vi "Stop Sequence.vi"(8 "error in (no error)":errorcluster, 11 "Connection Data In":T1) -> (0 "error out":errorcluster, 3 "Connection Data Out":T1)   [LabVIEW 2014, in "MSX-E3711_dll.lvlib"]
doc: "Detiene la Adquisición del modo Séquence."
uses:
  MSX-E3711_dll.lvlib
  Typedef/Connection Data.ctl
  E:/Repositorio Magnis/INF002/v0/Modules/HAL/Drivers/Sync/ADDI-DATA MSX-E3711/API/MSXE371x.dll
  MSXE371x.dll
  E:/Repositorio Magnis/INF002/v0/Modules/HAL/Drivers/Sync/ADDI-DATA MSX-E3711/API/MXCommon.dll
  MXCommon.dll
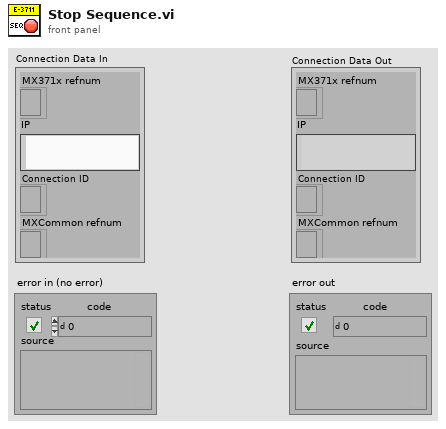
[diagram p1: front panel]
types:
  T1 = typedef "MSX-E3711_dll.lvlib/Connection Data.ctl" = cluster{"MX371x refnum":refnum<k24>, "IP":string, "Connection ID ":refnum<k5>, "MXCommon refnum":refnum<k24>}
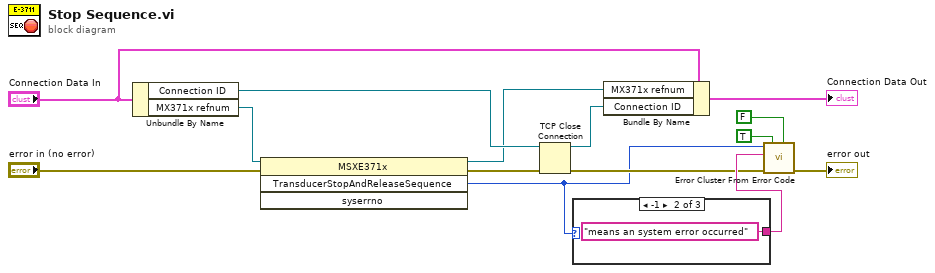
[diagram p0: block diagram]
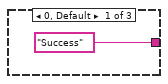
[diagram p2: hidden frame]
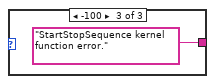
[diagram p3: hidden frame]
diagram:
  n1 = Unbundle By Name("Connection Data In") -> ("Connection ID"=w8:refnum<k5>, "MX371x refnum"=w6:refnum<k24>)
  n2 = invoke class="MSXE371x" method="TransducerStopAndReleaseSequence"(reference=w6, error in="error in (no error)") -> (reference out=w5:refnum<k24>, error out=w4:errorcluster, "TransducerStopAndReleaseSequence"=w3:i32)  [unwired: 2 in, 1 out]
  n3 = TCP Close Connection(connection ID=w8, error in (no error)=w4) -> (connection ID out=w7:refnum<k5>, error out=w9:errorcluster)  [unwired: 1 in]
  n4 = case shown="-1" w3 {
    tunnel: ["Success" "means an system error occurred" "StartStopSequence kernel function error."] -> w12
    frame 0, Default {
    }
    frame -1 {
    }
    frame -100 {
    }
  }
  n5 = Bundle By Name(cluster="Connection Data In", "MX371x refnum"=w5, "Connection ID"=w7) -> (→"Connection Data Out":T1)
  n6 = call <vilib>:"Error Cluster From Error Code.vi"("is warning? (False)"=FALSE, "show call chain? (False)"=TRUE, "error in (no error)"=w9, "error message (\"\")"=w12, "error code (0)"=w3) -> ("error out"=→"error out":errorcluster)  [unwired: 4 in]
